vi "OAT Check Overlap of Rectangles.vi"(5 "rect 2":T1, 7 "rect 1":T1) -> (2 "overlap":bool)   [LabVIEW 2017]
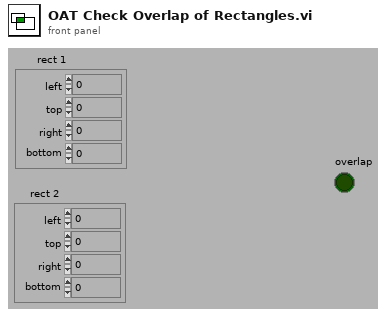
[diagram p1: front panel]
types:
  T1 = cluster{"left":i16, "top":i16, "right":i16, "bottom":i16}
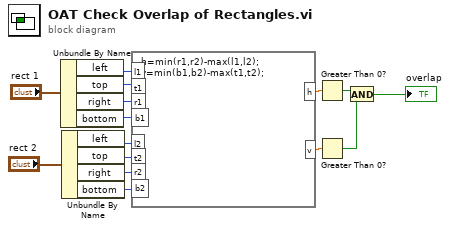
[diagram p0: block diagram]
diagram:
  n1 = Unbundle By Name("rect 1") -> ("left"=w13:i16, "top"=w12:i16, "right"=w11:i16, "bottom"=w10:i16)
  n2 = Unbundle By Name("rect 2") -> ("left"=w9:i16, "top"=w8:i16, "right"=w7:i16, "bottom"=w6:i16)
  n3 = formula code="h=min(r1,r2)-max(l1,l2);\nv=min(b1,b2)-max(t1,t2);"("l1"=w13, "t1"=w12, "r1"=w11, "b1"=w10, "l2"=w9, "t2"=w8, "r2"=w7, "b2"=w6) -> ("h"=w5:dbl, "v"=w4:dbl)
  n4 = Greater Than 0?(x=w5) -> (x > 0?=w3:bool)
  n5 = Greater Than 0?(x=w4) -> (x > 0?=w2:bool)
  n6 = And(x=w3, y=w2) -> (x .and. y?=→"overlap":bool)
